vi "Zad2.vi"() -> ()   [LabVIEW 2015]
uses:
  Control 1.ctl
panel:
  in  "stop":bool
  out "Waveform Chart":dbl(graph)
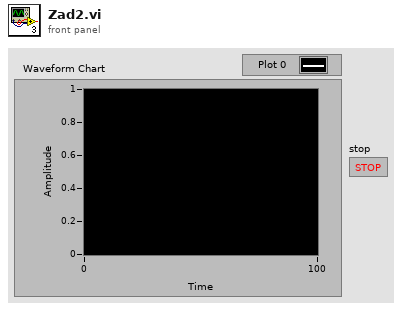
[diagram p1: front panel]
types:
  T1 = typedef "Control 1.ctl" = enum16{"Pomiar", "Wybór", "Eksport", "Zamkniecie"}
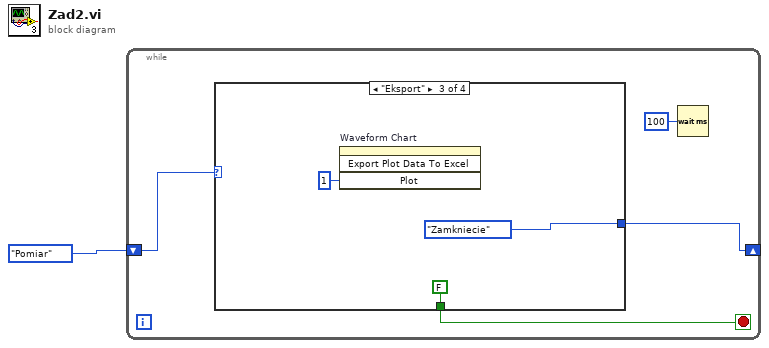
[diagram p0: block diagram]
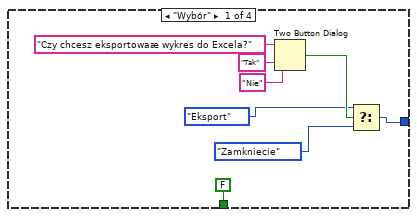
[diagram p2: hidden frame]
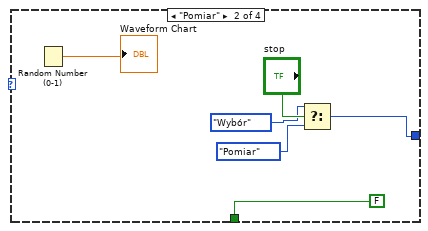
[diagram p3: hidden frame]
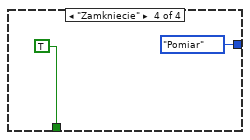
[diagram p4: hidden frame]
diagram:
  n1 = while {
    shift-right: [w2] -> _
    shift-left: Control_1."Pomiar" -> [w5]
    stop <- w4 stop-if-true
    n2 = case shown="\"Eksport\"" w5 {
      tunnel: [w9 w14 Control_1."Zamkniecie" ("f") Control_1."Pomiar" ("f")] -> w2
      tunnel: [FALSE FALSE FALSE TRUE] -> w4
      frame "Wybór" {
        n3 = Two Button Dialog(message="Czy chcesz eksportowaæ wykres do Excela?", 1:"Nie" ("F button name (\"Cancel\")"), 2:"Tak" ("T button name (\"OK\")")) -> (T button?=w10:bool)
        n4 = Select(t=Control_1."Eksport", s=w10, f=Control_1."Zamkniecie") -> (s? t:f=w9:T1)
      }
      frame "Pomiar" {
        n5 = Random Number (0-1)() -> (number: 0 to 1=→"Waveform Chart":dbl)
        n6 = Select(t=Control_1."Wybór", s="stop", f=Control_1."Pomiar") -> (s? t:f=w14:T1)
      }
      frame "Eksport" {
        n7 = invoke on="Waveform Chart" class="WFChart (strict)" method="Export Plot Data To Excel"("Plot"=1) -> ()  [unwired: 3 in, 4 out]
      }
      frame "Zamkniecie" {
      }
    }
    n8 = Wait (ms)(milliseconds to wait=u32 100) -> ()  [unwired: 1 out]
  }
